vi "TTC image manipulation.vi"(0 "Image in":T1, 1 "OIS image resolution":i32[](array[numeric]), 2 "TTC image resolution":i32[](array[numeric]), 5 "TTC vertical reverse":bool caption="Vertical reverse", 7 "TTC horizontal reverse":bool caption="Horizontal reverse", 9 "center X":u32(slide)=640 scale=0.0..640.0, 11 "center Y":u32(slide)=471, 12 "TTC Zoom":dbl(slide)=0.23059004545211792 caption="Zoom" scale=0.001..1.0, 13 "error in (no error)":errorcluster) -> (4 "Image out":T1, 6 "image center out":cluster{"X":u32, "Y":u32}, 8 "Zoom":cluster{"X":sgl, "Y":sgl}, 14 "error out":errorcluster)   [LabVIEW 2012]
uses:
  <vilib>/vision/Image Controls.llb/IMAQ Image.ctl
  <vilib>/vision/NI_Vision_Development_Module.lvlib
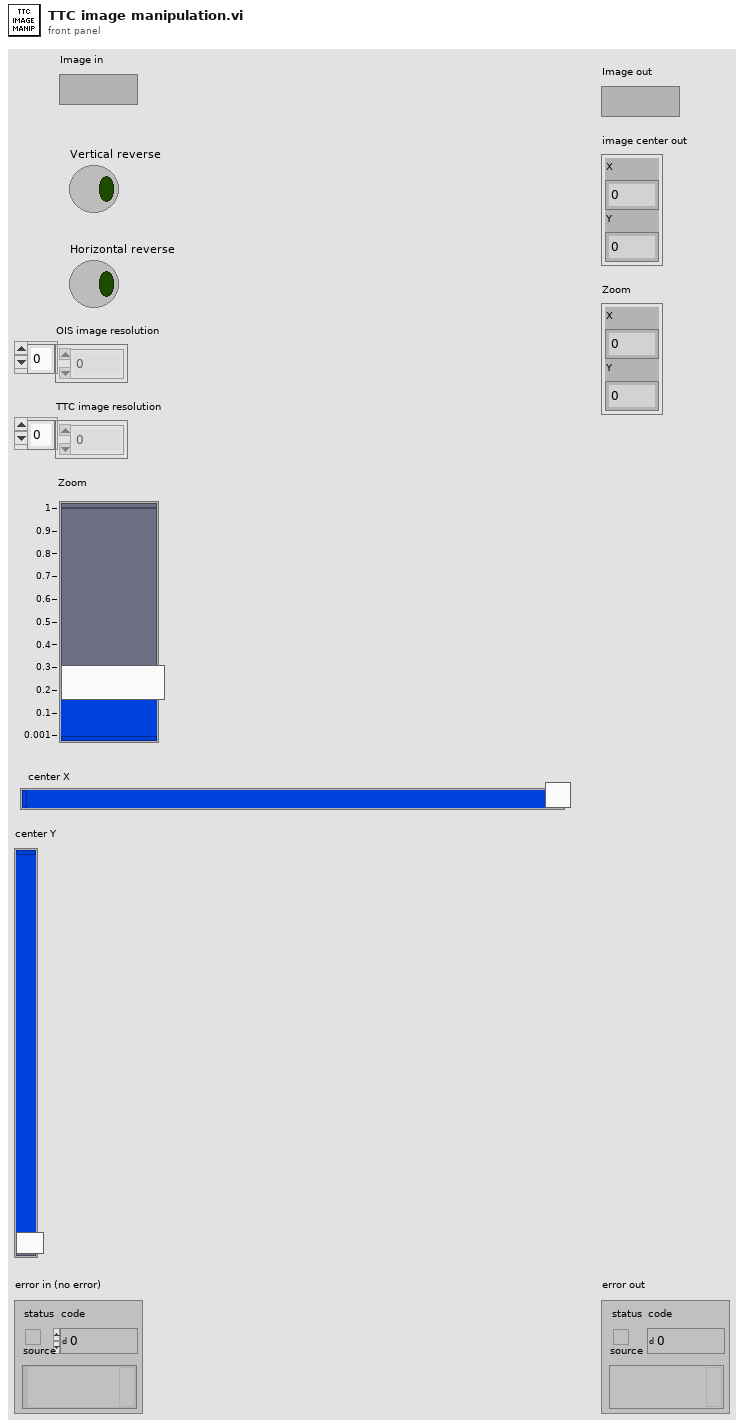
[diagram p1: front panel]
types:
  T1 = typedef "IMAQ Image.ctl" = refnum<image>
  T2 = typedef "Image Type" = u32
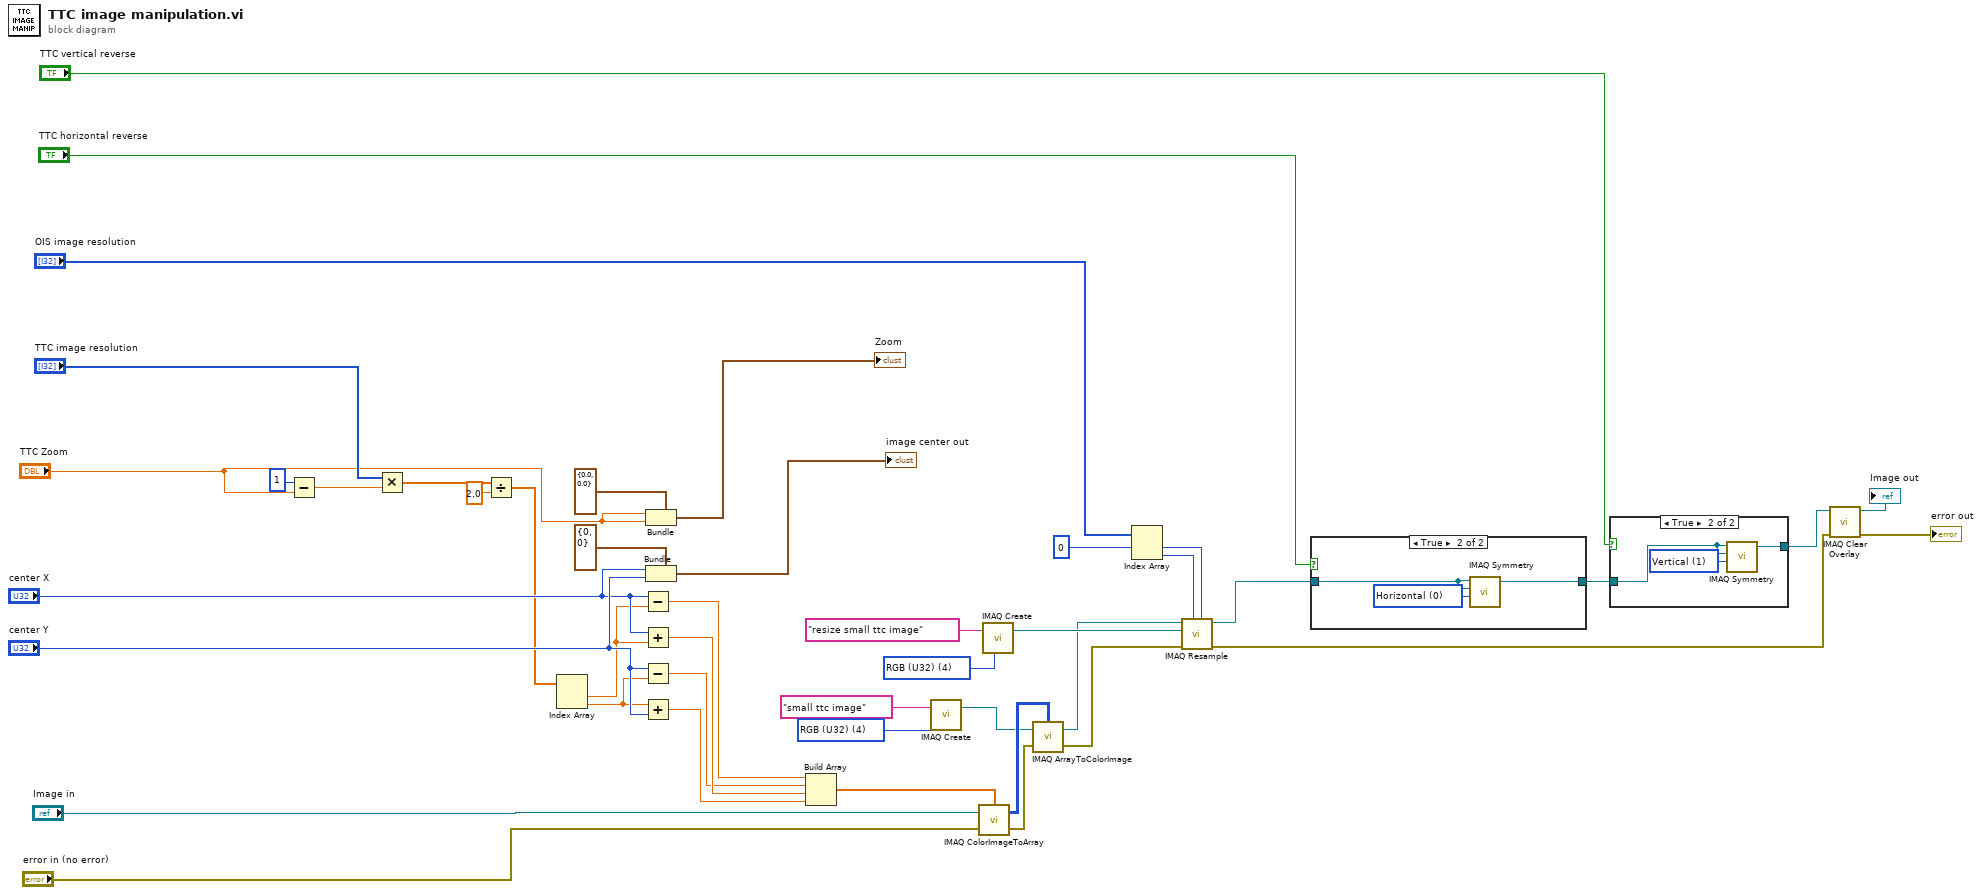
[diagram p0: block diagram]
diagram:
  w20 = T2 4 items=["Grayscale (U8)", "Grayscale (I16)", "Grayscale (SGL)", "Complex (CSG)", "RGB (U32)", "HSL (U32)", "RGB (U64)", "Grayscale (U16)"] ("Image Type")
  w2 = T2 4 items=["Grayscale (U8)", "Grayscale (I16)", "Grayscale (SGL)", "Complex (CSG)", "RGB (U32)", "HSL (U32)", "RGB (U64)", "Grayscale (U16)"] ("Image Type")
  n1 = Subtract(x=1, y="TTC Zoom") -> (x-y=w15:dbl)
  n2 = Multiply(x="TTC image resolution", y=w15) -> (x*y=w13:dbl[])
  n3 = Divide(x=w13, y=2.0 ("Zoom")) -> (x/y=w16:dbl[])
  n4 = Index Array(array=w16) -> (element #1=w8:dbl, element #2=w9:dbl)  [unwired: 2 in]
  n5 = Subtract(x="center X", y=w8) -> (x-y=w7:dbl)
  n6 = Add(x="center X", y=w8) -> (x+y=w10:dbl)
  n7 = Subtract(x="center Y", y=w9) -> (x-y=w6:dbl)
  n8 = Add(x=w9, y="center Y") -> (x+y=w11:dbl)
  n9 = Bundle(cluster=cluster{"X":sgl, "Y":sgl} {"X"=0.0, "Y"=0.0} ("ZoomSingle:All Elements"), "X"="TTC Zoom", "Y"="TTC Zoom") -> (→"Zoom":cluster{"X":sgl, "Y":sgl})
  n10 = Bundle(cluster=cluster{"X":u32, "Y":u32} {"X"=0, "Y"=0} ("Center Position"), "X"="center X", "Y"="center Y") -> (→"image center out":cluster{"X":u32, "Y":u32})
  n11 = Build Array(w7, w6, w10, w11) -> (w12:dbl[])
  n12 = call "IMAQ Create"("Image Name"="small ttc image", "Image Type"=w2) -> ("New Image"=w3:T1)  [unwired: 3 in, 1 out]
  n13 = call "IMAQ ColorImageToArray"("Optional Rectangle"=w12, "Image"="Image in", "error in (no error)"="error in (no error)") -> ("Image Pixels (U32)"=w4:u32[][], "error out"=w31:errorcluster)  [unwired: 1 in, 1 out]
  n14 = call "IMAQ Create"("Image Name"="resize small ttc image", "Image Type"=w20) -> ("New Image"=w22:T1)  [unwired: 3 in, 1 out]
  n15 = call "IMAQ ArrayToColorImage"("Image Pixels (U32)"=w4, "Image"=w3, "error in (no error)"=w31) -> ("Image Out"=w19:T1, "error out"=w32:errorcluster)  [unwired: 2 in]
  n16 = Index Array(array="OIS image resolution", index #1=0 ("index")) -> (element #1=w37:i32, element #2=w38:i32)  [unwired: 1 in]
  n17 = call "IMAQ Resample"("X Resolution"=w37, "Y Resolution"=w38, "error in (no error)"=w32, "Image Dst"=w22, "Image Src"=w19) -> ("error out"=w33:errorcluster, "Image Dst Out"=w23:T1)  [unwired: 5 in]
  n18 = case shown="True" "TTC horizontal reverse" {
    tunnel: w23 -> [w45 w47]
    tunnel: [w45 w46] -> w24
    frame False {
    }
    frame True {
      w48 = u32 0 items=["Horizontal", "Vertical", "Central", "1st Diagonal", "2nd Diagonal"] ("Type of Symmetry")
      n19 = call "IMAQ Symmetry"("Type of Symmetry"=w48, "Image Dst"=w47, "Image Src"=w47) -> ("Image Dst Out"=w46:T1)  [unwired: 2 in, 1 out]
    }
  }
  n20 = case shown="True" "TTC vertical reverse" {
    tunnel: w24 -> [w49 w52]
    tunnel: [w49 w50] -> w30
    frame False {
    }
    frame True {
      w51 = u32 1 items=["Horizontal", "Vertical", "Central", "1st Diagonal", "2nd Diagonal"] ("Type of Symmetry")
      n21 = call "IMAQ Symmetry"("Type of Symmetry"=w51, "Image Dst"=w52, "Image Src"=w52) -> ("Image Dst Out"=w50:T1)  [unwired: 2 in, 1 out]
    }
  }
  n22 = call "IMAQ Clear Overlay"("error in (no error)"=w33, "Image"=w30) -> ("error out"=→"error out":errorcluster, "Image Out"=→"Image out":T1)  [unwired: 8 in]
